vi "ControlPathToArray.vi"(0 "Control Name":string, 1 "delimiter (>>)":string) -> (2 "Control Path":string[](array[string]))   [LabVIEW 2016]
doc: "Converts control path to array"
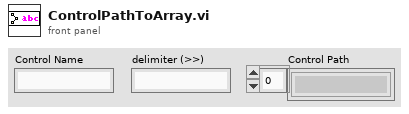
[diagram p1: front panel]
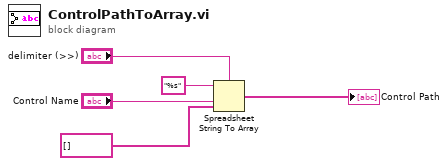
[diagram p0: block diagram]
diagram:
  n1 = Spreadsheet String To Array(delimiter (Tab)="delimiter (>>)", format string="%s", spreadsheet string="Control Name", array type (2D Dbl)=string[] []) -> (array=→"Control Path":string[])
